vi "실습 7-4.vi"() -> ()   [LabVIEW 2014]
panel:
  out "array":dbl[](array[numeric])
  in  "filePath":string
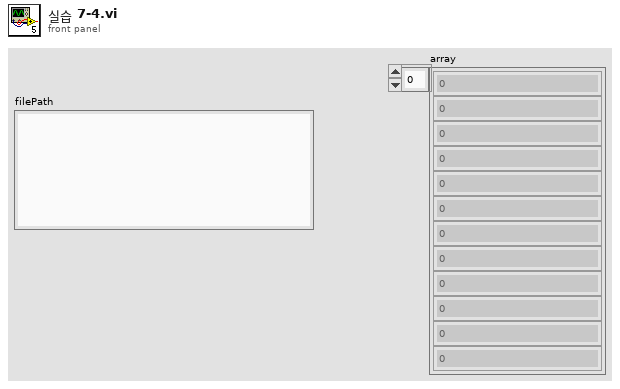
[diagram p1: front panel]
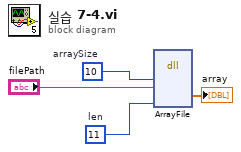
[diagram p0: block diagram]
diagram:
  w4 = 10  # arraySize
  w2 = 11  # len
  n1 = dll-call lib="PTH2\\abs CUserslveduDesktop중급 LabVIEWbuilds\tDLL실습\n나의 DLL\nSharedLib.dll" fn="ArrayFile"("arraySize"=w4, "filePath"="filePath", "len"=w2) -> ("array"=→"array":dbl[])  [unwired: 8 in, 2 out]
